vi "ACP Configure Carrier Channel.vi"(7 "Selector String":string, 8 "error in (no error)":errorcluster, 10 "ACP Carrier Channel Configuration":T1=[{"Carrier Frequency (Hz)"=0.0, "Integration Bandwidth (Hz)"=18000000.0, "RRC Filter"={"Alpha"=0.22, "Enabled"=0}, "Mode"=1}] {"Mode" items=["Passive", "Active"]; "Carrier Frequency (Hz)" format="%.3p"; "RRC Filter"."Enabled" items=["False", "True"]; "RRC Filter"."Alpha" format="%.3g"; "Integration Bandwidth (Hz)" format="%.3p"}, 11 "Instrument Handle In":refnum<k21>) -> (0 "error out":errorcluster, 3 "Instrument Handle Out":refnum<k21>)   [LabVIEW 2016, in "RFmxSpecAn.lvlib"]
uses:
  RFmxSpecAn.lvlib
  Typedefs/ACP Carrier Channel Configuration.ctl
  <vilib>/RFmx/SpecAn/mx/RFmxSpecAn.llb/RFmxSpecAn Build Signal String.vi
  <vilib>/RFmx/RFInstr/mx/RFmxInstr.llb/RFmxInstr Build Signal String.vi
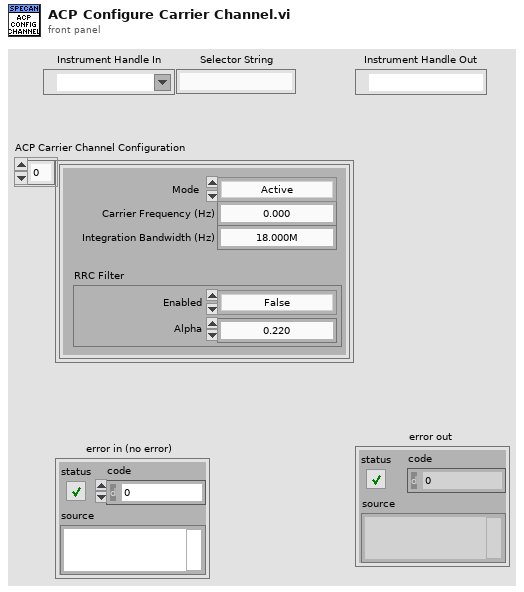
[diagram p1: front panel]
types:
  T1 = typedef "RFmxSpecAn.lvlib/ACP Carrier Channel Configuration.ctl" = cluster{"Carrier Frequency (Hz)":dbl, "Integration Bandwidth (Hz)":dbl, "RRC Filter":cluster{"Alpha":dbl, "Enabled":i32}, "Mode":i32}[]
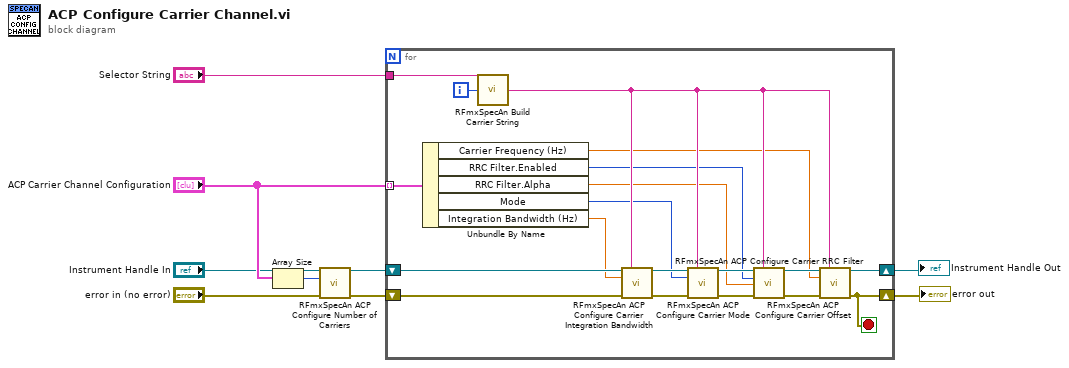
[diagram p0: block diagram]
diagram:
  n1 = Array Size(array="ACP Carrier Channel Configuration") -> (size(s)=w7:i32)
  n2 = call <vilib>:"RFmxSpecAn ACP Configure Number of Carriers.vi"("Instrument Handle In"="Instrument Handle In", "Number of Carriers"=w7, "error in (no error)"="error in (no error)") -> ("Instrument Handle Out"=w9:refnum<k21>, "error out"=w8:errorcluster)  [unwired: 11 in]
  n3 = for {
    tunnel: "ACP Carrier Channel Configuration" -> [w20] mode=indexing
    shift-right: [w16] -> w1
    shift-left: w8 -> [w27]
    shift-right: [w19] -> w2
    shift-left: w9 -> [w28]
    tunnel: "Selector String" -> [w10]
    i -> [w18]
    stop <- w16 stop-if-true
    n4 = Unbundle By Name(w20) -> ("Carrier Frequency (Hz)"=w15:dbl, "RRC Filter.Enabled"=w14:i32, "RRC Filter.Alpha"=w13:dbl, "Mode"=w12:i32, "Integration Bandwidth (Hz)"=w11:dbl)
    n5 = call <vilib>:"RFmxSpecAn Build Carrier String.vi"("Signal Name"=w10, "Carrier Number"=w18) -> ("Carrier String"=w17:string)  [unwired: 13 in]
    n6 = call <vilib>:"RFmxSpecAn ACP Configure Carrier Integration Bandwidth.vi"("Instrument Handle In"=w28, "Selector String"=w17, "Integration Bandwidth (Hz)"=w11, "error in (no error)"=w27) -> ("Instrument Handle Out"=w26:refnum<k21>, "error out"=w25:errorcluster)  [unwired: 10 in]
    n7 = call <vilib>:"RFmxSpecAn ACP Configure Carrier Mode.vi"("Instrument Handle In"=w26, "Selector String"=w17, "Carrier Mode"=w12, "error in (no error)"=w25) -> ("Instrument Handle Out"=w24:refnum<k21>, "error out"=w23:errorcluster)  [unwired: 10 in]
    n8 = call <vilib>:"RFmxSpecAn ACP Configure Carrier RRC Filter.vi"("Instrument Handle In"=w24, "Selector String"=w17, "RRC Filter Enabled"=w14, "RRC Alpha"=w13, "error in (no error)"=w23) -> ("Instrument Handle Out"=w22:refnum<k21>, "error out"=w21:errorcluster)  [unwired: 9 in]
    n9 = call <vilib>:"RFmxSpecAn ACP Configure Carrier Offset.vi"("Instrument Handle In"=w22, "Selector String"=w17, "Carrier Frequency (Hz)"=w15, "error in (no error)"=w21) -> ("Instrument Handle Out"=w19:refnum<k21>, "error out"=w16:errorcluster)  [unwired: 10 in]
  }
  "Instrument Handle Out" <- w2
  "error out" <- w1
